vi "Animation.vi"() -> ()   [LabVIEW 2018]
uses:
  FGV/FGV_mods.ctl
  <vilib>/Heliosphere Research LLC/Advanced Plotting Toolkit/api_core/NewPlotType.ctl
  <vilib>/Analysis/1siggen.llb/Ramp Pattern by Samples.vi
  <vilib>/Analysis/NI_AALBase.lvlib
  <vilib>/Heliosphere Research LLC/Advanced Plotting Toolkit/Advanced Plotting Toolkit.lvlib
panel:
  in  "max_cont":i32=100 caption="Max cont"
  in  "hits":i32=100 caption="Hits per frame"
  in  "dir_pics":path caption="Directory pictures"
  out "Progresso":dbl(slide) scale=0.0..100.0
  in  "Channel":i32=1
  out "error out":errorcluster
  out "Polar":picture
  in  "file":path caption="Directory tests"
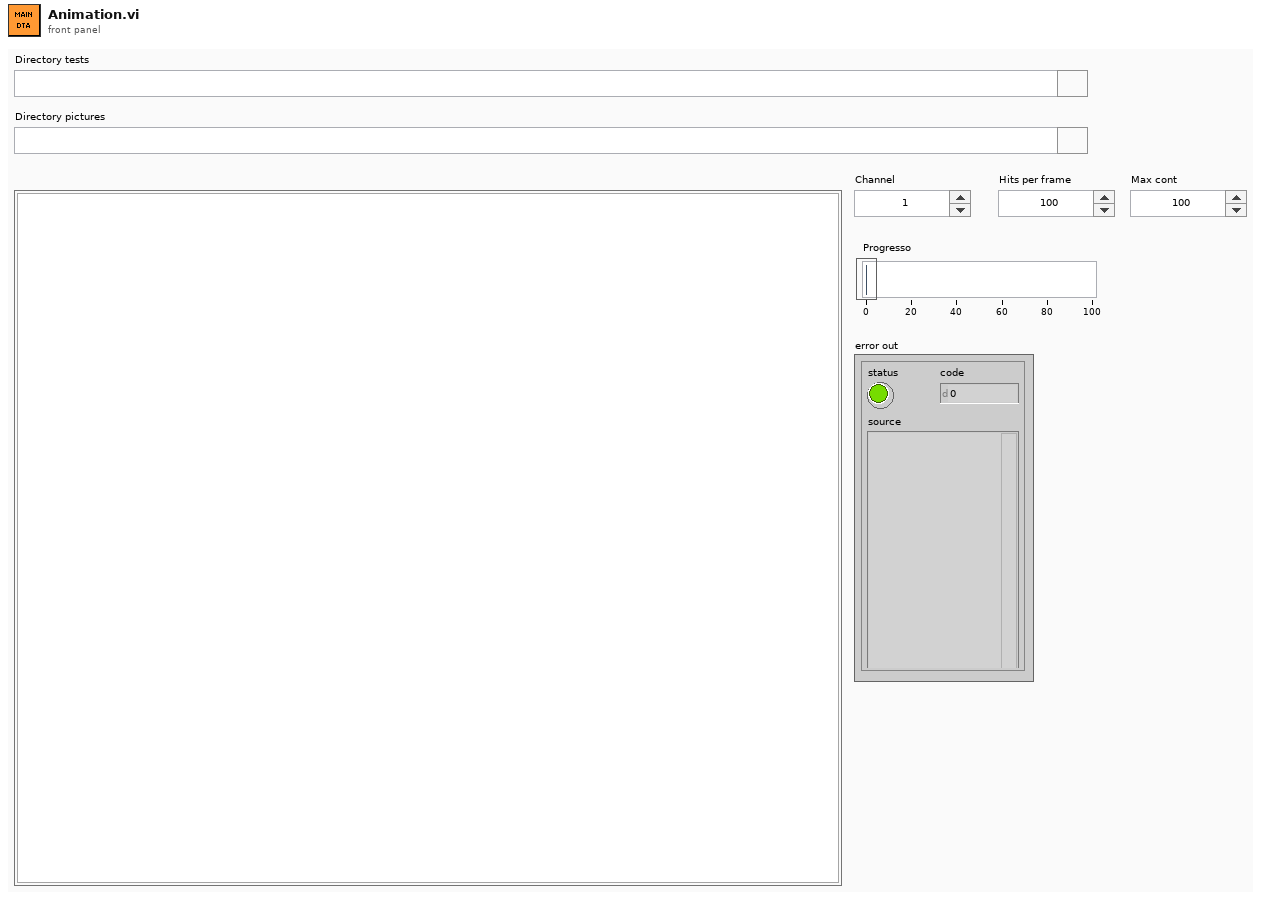
[diagram p1: front panel]
types:
  T1 = typedef "FGV_mods.ctl" = enum16{"Init", "get_config", "get_hits", "set_file", "open_file", "get_startTime", "close"}
  T2 = typedef "Advanced Plotting Toolkit.lvlib/NewPlotType.ctl" = enum16{"Rectangular Axes", "Polar Axes"}
  T3 = typedef "hit_data.ctl" = cluster{"channel":u8, "time":dbl, "parameters":cluster{"riseTime":u32, "countsToPeak":u32, "counts":u32, "energy":u32, "duration":u32, "amplitude":u32, "RMS":u32, "ASL":u32, "gain":u32, "THR":u32, "preAmp":u32, "avrFreq":u32}}
  T4 = typedef "polar_data.ctl" = cluster{"t0":dbl, "conts":dbl[], "amps":dbl[]}
  T5 = typedef "Advanced Plotting Toolkit.lvlib/PlotID.ctl" = i32
  T6 = typedef "imagedata.ctl" = cluster{"image type":i32, "image depth":i32, "image":u8[], "mask":u8[], "colors":u32[], "Rectangle":cluster{"left":i16, "top":i16, "right":i16, "bottom":i16}}
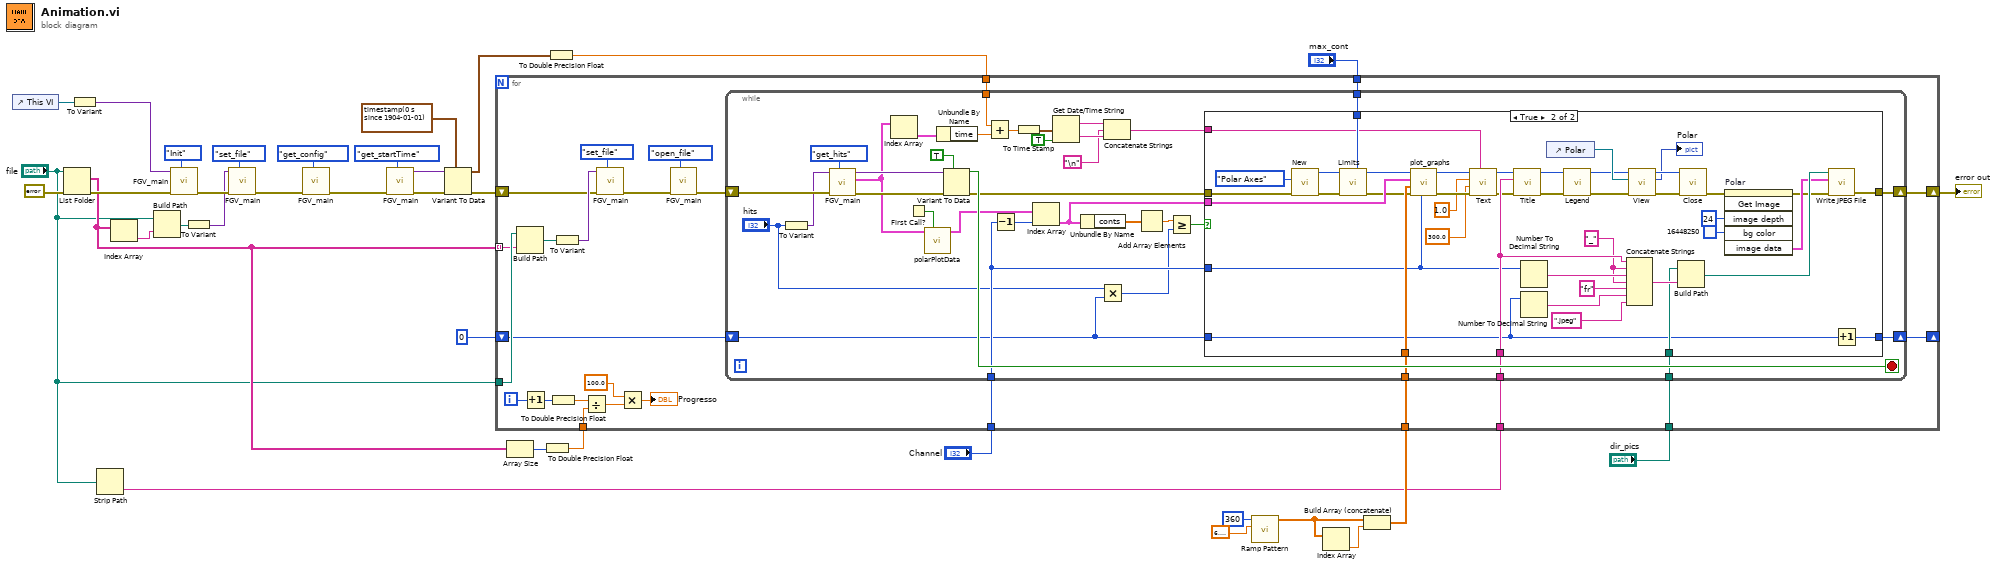
[diagram p0: block diagram]
diagram:
  n1 = control-ref of="This VI"() -> (w35:refnum<vi>)
  n2 = List Folder(path="file", error in=errorcluster {"status"=FALSE, "code"=0, "source"=""} ("Error Out")) -> (filenames=w23:string[], error out=w27:errorcluster)  [unwired: 2 in, 2 out]
  n3 = To Variant(anything=w35) -> (Variant=w28:variant)
  n4 = Strip Path(path="file") -> (name=w12:string)  [unwired: 1 out]
  n5 = Index Array(array=w23) -> (element=w33:string)  [unwired: 1 in]
  n6 = Build Path(base path="file", name or relative path=w33) -> (appended path=w32:path)
  n7 = call "FGV_main.vi"("FGV_mods"=FGV_mods."Init", "Error In"=w27, "DataIn"=w28) -> ("Error Out"=w31:errorcluster)  [unwired: 6 in, 2 out]
  n8 = To Variant(anything=w32) -> (Variant=w24:variant)
  n9 = call "FGV_main.vi"("FGV_mods"=FGV_mods."set_file", "Error In"=w31, "DataIn"=w24) -> ("Error Out"=w25:errorcluster)  [unwired: 6 in, 2 out]
  n10 = call "FGV_main.vi"("FGV_mods"=FGV_mods."get_config", "Error In"=w25) -> ("Error Out"=w7:errorcluster)  [unwired: 7 in, 2 out]
  n11 = call "FGV_main.vi"("FGV_mods"=FGV_mods."get_startTime", "Error In"=w7) -> ("Error Out"=w5:errorcluster, "DataOut"=w6:variant)  [unwired: 7 in, 1 out]
  n12 = Variant To Data(error in=w5, type=timestamp(0 s since 1904-01-01), Variant=w6) -> (data=w2:timestamp, error out=w4:errorcluster)
  n13 = Array Size(array=w23) -> (size(s)=w22:i32)
  n14 = To Double Precision Float(number=w22) -> (double precision float=w21:dbl)
  n15 = To Double Precision Float(number=w2) -> (double precision float=w1:dbl)
  n16 = call-poly <vilib>:"Ramp Pattern.vi"("end"=6.283185307179586, "samples"=360) -> ("Ramp Pattern"=w16:dbl[])  [unwired: 8 in, 1 out]
  n17 = Index Array(array=w16) -> (element=w17:dbl)  [unwired: 1 in]
  n18 = Build Array (concatenate)(w16, w17) -> (w14:dbl[])
  n19 = for {
    shift-right: [w40] -> w11
    shift-left: w4 -> [w52]
    tunnel: "file" -> [w56]
    tunnel: w23 -> [w55] mode=indexing
    tunnel: w21 -> [w48]
    tunnel: "Channel" -> [w44]
    tunnel: w14 -> [w43]
    tunnel: "dir_pics" -> [w42]
    tunnel: w12 -> [w41]
    shift-right: [w38] -> _
    shift-left: 0 -> [w39]
    tunnel: "max_cont" -> [w37]
    tunnel: w1 -> [w36]
    i -> [w51]
    n20 = Build Path(base path=w56, name or relative path=w55) -> (appended path=w54:path)
    n21 = Increment(x=w51) -> (x+1=w50:i32)
    n22 = To Double Precision Float(number=w50) -> (double precision float=w49:dbl)
    n23 = To Variant(anything=w54) -> (Variant=w53:variant)
    n24 = Divide(x=w49, y=w48) -> (x/y=w47:dbl)
    n25 = call "FGV_main.vi"("FGV_mods"=FGV_mods."set_file", "Error In"=w52, "DataIn"=w53) -> ("Error Out"=w57:errorcluster)  [unwired: 6 in, 2 out]
    n26 = Multiply(x=100.0, y=w47) -> (x*y=→"Progresso":dbl)
    n27 = call "FGV_main.vi"("FGV_mods"=FGV_mods."open_file", "Error In"=w57) -> ("Error Out"=w59:errorcluster)  [unwired: 7 in, 2 out]
    n28 = while {
      shift-right: [w81] -> w40
      shift-left: w59 -> [w95]
      tunnel: w44 -> [w84]
      tunnel: w43 -> [w87]
      tunnel: w42 -> [w86]
      tunnel: w41 -> [w85]
      shift-right: [w76] -> w38
      shift-left: w39 -> [w75]
      tunnel: w37 -> [w72]
      tunnel: w36 -> [w69]
      stop <- w91 stop-if-true
      n29 = To Variant(anything="hits") -> (Variant=w94:variant)
      n30 = call "FGV_main.vi"("FGV_mods"=FGV_mods."get_hits", "Error In"=w95, "DataIn"=w94) -> ("Error Out"=w89:errorcluster, "hits"=w71:T3[], "DataOut"=w93:variant)  [unwired: 6 in]
      n31 = Index Array(array=w71) -> (element=w70:T3)  [unwired: 1 in]
      n32 = First Call?() -> (First Call?: T/F=w90:bool)
      n33 = call "polarPlotData.vi"("reset"=w90, "hits"=w71) -> ("polar_plot_data"=w83:T4[])  [unwired: 9 in]
      n34 = Unbundle By Name(w70) -> ("time"=w68:dbl)
      n35 = Variant To Data(error in=w89, type=TRUE, Variant=w93) -> (data=w91:bool, error out=w82:errorcluster)
      n36 = Add(x=w69, y=w68) -> (x+y=w67:dbl)
      n37 = Decrement(x=w84) -> (x-1=w88:i32)
      n38 = To Time Stamp(1:w67) -> (0:w66:timestamp)
      n39 = Index Array(array=w83, index=w88) -> (element=w80:T4)
      n40 = Get Date/Time String(seconds (now)=w66, want seconds? (F)=TRUE) -> (date string=w63:string, time string=w64:string)  [unwired: 1 in]
      n41 = Unbundle By Name(w80) -> ("conts"=w79:dbl[])
      n42 = Multiply(x="hits", y=w75) -> (x*y=w73:i32)
      n43 = Concatenate Strings(w63, "\n", w64) -> (w62:string)
      n44 = Add Array Elements(numeric array=w79) -> (sum=w78:dbl)
      n45 = Greater Or Equal?(x=w78, y=w73) -> (x >= y?=w77:bool)
      n46 = case shown="True" w77 {
        tunnel: w87 -> [_ w126]
        tunnel: w86 -> [_ w125]
        tunnel: w85 -> [_ w124]
        tunnel: w84 -> [_ w120]
        tunnel: w82 -> [w98 w119]
        tunnel: [w98 w118] -> w81
        tunnel: w80 -> [_ w114]
        tunnel: w75 -> [w97 w112]
        tunnel: [w97 w113] -> w76
        tunnel: w72 -> [_ w106]
        tunnel: w62 -> [_ w101]
        frame False {
        }
        frame True {
          w117 = "_" ("string")
          n47 = call <vilib>:"New.vi"("error in (no error)"=w119, "Plot Type"=NewPlotType."Polar Axes") -> ("error out"=w110:errorcluster, "Plot ID"=w107:T5)  [unwired: 8 in]
          n48 = call <vilib>:"Limits.vi"("Y Max"=w106, "error in (no error)"=w110, "Plot ID"=w107) -> ("error out"=w109:errorcluster, "Plot ID Out"=w108:T5)  [unwired: 7 in]
          n49 = call "plot_graphs.vi"("channel"=w120, "error in"=w109, "angs"=w126, "polar_data"=w114, "Plot ID"=w108) -> ("error out"=w105:errorcluster, "Plot ID out"=w102:T5)  [unwired: 5 in]
          n50 = call <vilib>:"Text.vi"("Text"=w101, "error in (no error)"=w105, "Y Position"=300.0 ("X Position"), "X Position"=1.0, "Plot ID"=w102) -> ("error out"=w104:errorcluster, "Plot ID Out"=w103:T5)  [unwired: 5 in]
          n51 = call <vilib>:"Title.vi"("error in (no error)"=w104, "Title"=w124, "Plot ID"=w103) -> ("error out"=w136:errorcluster, "Plot ID out"=w137:T5)  [unwired: 7 in]
          n52 = Number To Decimal String(number=w120) -> (decimal integer string=w138:string)  [unwired: 1 in]
          n53 = Number To Decimal String(number=w112) -> (decimal integer string=w111:string)  [unwired: 1 in]
          n54 = control-ref of="Polar"() -> (w129:refnum<vi>)
          n55 = call <vilib>:"Legend.vi"("error in (no error)"=w136, "Plot ID"=w137) -> ("error out"=w128:errorcluster, "Plot ID Out"=w127:T5)  [unwired: 8 in]
          n56 = Concatenate Strings(w124, w117, w138, w117, "fr" ("string"), w111, ".jpeg" ("string")) -> (w139:string)
          n57 = call <vilib>:"View.vi"("error in (no error)"=w128, "Ref for Sizing"=w129, "Plot ID"=w127) -> ("error out"=w131:errorcluster, "Picture"=→"Polar":picture, "Plot ID Out"=w132:T5)  [unwired: 6 in]
          n58 = Build Path(base path=w125, name or relative path=w139) -> (appended path=w140:path)
          n59 = call <vilib>:"Close.vi"("error in (no error)"=w131, "Plot ID"=w132) -> ("error out"=w133:errorcluster)  [unwired: 9 in]
          n60 = invoke on="Polar" class="Pict" method="Get Image"(error in=w133, "image depth"=24 ("Image Depth"), "bg color"=u32 16448250) -> (error out=w134:errorcluster, "image data"=w135:T6)  [unwired: 3 in, 4 out]
          n61 = call <vilib>:"Write JPEG File.vi"("error in (no error)"=w134, "image data"=w135, "path to JPEG file"=w140) -> ("error out"=w118:errorcluster)  [unwired: 7 in, 1 out]
          n62 = Increment(x=w112) -> (x+1=w113:i32)
        }
      }
    }
  }
  "error out" <- w11
